vi "PH_Synchrolock_Watch.panel.vi"(0 "object ref":refnum<vi>, 5 "error in (no error)":errorcluster) -> (19 "error out":errorcluster)   [LabVIEW 2014, in "PH_Synchrolock_Watch.lvlib"]
doc: "This a GUI.\n\nLicense Agreement for this software:\n\nCopyright (C)\nGesellschaft für Schwerionenforschung, GSI\nPlanckstr. 1\n64291 Darmstadt\nGermany\n\nContact: D.Beck@gsi.de \n\nThis program is free software; you can redistribute it and/or modify it under the terms of the GNU General Public License as published by the Free Software Foundation; either version 2 of the license, or (at your option) any later version.\n\nThis program is distributed in the hope that it will be useful, but WITHOUT ANYW ARRANTY; without even the implied warranty of MERCHANTABILITY or FITNESS FOR A PARTICULAR PURPOSE. See the GNU General License for more details (http://www.gnu.org).\n\nGesellschaft für Schwerionenforschung, GSI\nPlanckstr. 1, 64291 Darmstadt, Germany\nFor all questions and ideas contact: M.Richter@gsi.de, H.Brand@gsi.de or D.Beck@gsi.de.\nLast update: 18-DEC-2002"
uses:
  PH_Synchrolock_Watch.lvlib
  PH_StatusHandler/PH_StatusHandler.GUI element.ctl
  PH_TKTDS-30xx/PH_TKTDS-30xx.Channel Config.ctl
  PH_TKTDS-30xx/PH_TKTDS-30xx.Acquisition Config.ctl
  PH_TKTDS-30xx/PH_TKTDS-30xx.Trigger Config.ctl
  PH_TKTDS-30xx/PH_TKTDS-30xx.GUI Refs.ctl
  PH_Synchrolock_Watch.Limit to set.ctl
  CSCore/CSObj/CSObj.lvlib
  PH_Common/PH_Common.lvlib
  CSCore/CSSystem/CSSystemLib/CSSystemLib.lvlib
  PH_TKTDS-30xx/PH_TKTDS-30xx.lvlib
  PH_Class/PH_Class.lvlib
  PH_StatusHandler/PH_StatusHandler.lvlib
panel:
  out "VISA Resource":string
  out "Dummy":waveform(dbl)[](graph)
  out "State":u32(colorbox)
  in  "Tab Control":T1(tab)
  in  "Waveform End":i32=10000
  out "MIRA State":u32(colorbox)
  out "Mira scope":cluster{dbl[], dbl[]}[](graph)=[{array[1000 elements], array[1000 elements]}, {array[1000 elements], array[1000 elements]}, {[7.678540433925049e-09, 2.168621418974559e-08, 3.532212428448502e-08, 4.8880103626943005e-08, 6.250409620353807e-08, 7.640981633945535e-08, 9.060849771566783e-08, 1.0463764927718417e-07, 1.1843036179225119e-07, 1.3205722912966255e-07, 1.456689870009999e-07, 1.593456671426305e-07, 1.733563575717145e-07, 1.8748672524777768e-07], [0.1328923695789544, 0.14553699894253908, 0.15804846129472974, 0.158480311601262, 0.15023324530868346, 0.13645178082078474, 0.12443003311658221, 0.1394555004984945, 0.1510217909126647, 0.15823883495688304, 0.1548392047127739, 0.14554396716656443, 0.1297955998863915, 0.1273963557283981]}, {[7.736674157303367e-09, 2.155081885856079e-08, 3.5410718232044194e-08, 4.9320659340659336e-08, 6.315258426966291e-08, 7.696082949308756e-08, 9.076550868486352e-08, 1.045925e-07, 1.1843617486338797e-07, 1.3226125e-07, 1.4617333333333334e-07, 1.6003049180327868e-07, 1.7381259259259259e-07, 1.87644e-07], [0.007461034259448418, 0.0073273846229039786, 0.007350860505608576, 0.006879176956376958, 0.007073457405515834, 0.007321165898617512, 0.0071646017369727056, 0.0071848909090909095, 0.007206295115085282, 0.007172368181818184, 0.007138666666666666, 0.007072396125186293, 0.007497003815937153, 0.007023602424242428]}]
  out "Mean Phase in range?":bool
  out "Mira Amplitude in range?":bool
  out "RF Amplitude above limit?":bool
  in  "Reset Mira warning":bool
  out "Mean Phase Graph":cluster{dbl[], dbl[]}[](graph) caption="Mean Phase"
  out "Mean Phase":dbl=2.090074050465849e-10 caption="Current Value" format="%^#_6e"
  in  "Mean phase upper limit":dbl=0.15 caption="Upper limit" format="%^#_6e"
  in  "Mean phase lower limit":dbl=-0.15 caption="Lower limit" format="%^#_6e"
  out "RF Amplitude Graph":cluster{dbl[], dbl[]}[](graph) caption="RF Amplitude"
  in  "RF Amplitude lower limit":dbl=0.13 caption="Lower limit" format="%^#_6e"
  out "RF Amplitude":dbl=0.14374031818040756 caption="Current Value" format="%^#_6e"
  out "Mira Amplitude Graph":cluster{dbl[], dbl[]}[](graph) caption="Mira Amplitude"
  in  "Mira Amplitude lower limit":dbl=0.0061 caption="Lower limit" format="%^#_6e"
  in  "Mira Amplitude upper limit":dbl=0.0068 caption="Upper limit" format="%^#_6e"
  out "Mira Amplitude":dbl=0.9056406758925662 caption="Current Value" format="%^#_6e"
  in  "Trigger":T2={"Source"="CH1", "Slope"=0, "Level [V]"=0.0} {"Level [V]" format="%#_6p"}
  in  "Acquisition":T3={"Time base"=2e-07, "Record Length"=10000, "Start Time"=0.0, "Type"=0, "Continuous"=FALSE} {"Start Time" format="%#_12p"; "Record Length" items=["500"=500, "10000"=10000]; "Time base" items=["2ns"=2e-09, "4ns"=4e-09, "10ns"=1e-08, "20ns"=2e-08, "40ns"=4e-08, "100ns"=1e-07, "200ns"=2e-07, "400ns"=4e-07, "1µs"=1e-06, "2µs"=2e-06, "4µs"=4e-06, "10µs"=1e-05, "20µs"=2e-05, "40µs"=4e-05, "100µs"=0.0001, "200µs"=0.0002, "400µs"=0.0004, "1ms"=0.001, "2ms"=0.002, "10ms"=0.01, "20ms"=0.02, "40ms"=0.04, "100ms"=0.1, "200ms"=0.2, "400ms"=0.4, "1s"=1.0, "2s"=2.0, "4s"=4.0, "10s"=10.0]}
  in  "Mira Signal":T4={"Channel Name"="CH1", "Input Impedance"="MEG", "Max Input Frequency"="TWENTY", "Vertical Coupling"=1, "Channel Enabled"=TRUE, "Probe Attenuation"=1.0, "Vertical Range"=100.0, "Vertical Offset"=0.0} {"Vertical Offset" format="%#_6p"; "Vertical Range" items=["1mV"=0.001, "2mV"=0.002, "5mV"=0.005, "10mV"=0.01, "20mV"=0.02, "50mV"=0.05, "100mV"=0.1, "200mV"=0.2, "500mV"=0.5, "1V"=1.0]; "Probe Attenuation" format="%#.2f"}
  in  "RF Signal":T4={"Channel Name"="CH1", "Input Impedance"="MEG", "Max Input Frequency"="TWENTY", "Vertical Coupling"=1, "Channel Enabled"=TRUE, "Probe Attenuation"=1.0, "Vertical Range"=100.0, "Vertical Offset"=0.0} {"Vertical Offset" format="%#_6p"; "Vertical Range" items=["1mV"=0.001, "2mV"=0.002, "5mV"=0.005, "10mV"=0.01, "20mV"=0.02, "50mV"=0.05, "100mV"=0.1, "200mV"=0.2, "500mV"=0.5, "1V"=1.0]; "Probe Attenuation" format="%#.2f"}
  in  "Display Intensity":u8=1 min=1 max=100 step=1
  in  "Channel to be positioned":string(combo)="CH1"
  in  "Position":dbl
  out "PSDB Status":u32(colorbox)=6618880 caption="PSDB"
  out "Status":T5 caption="Enabling State"
  in  "Delete":bool
  in  "Exit":bool
  # "PCS"
  # "3.40"
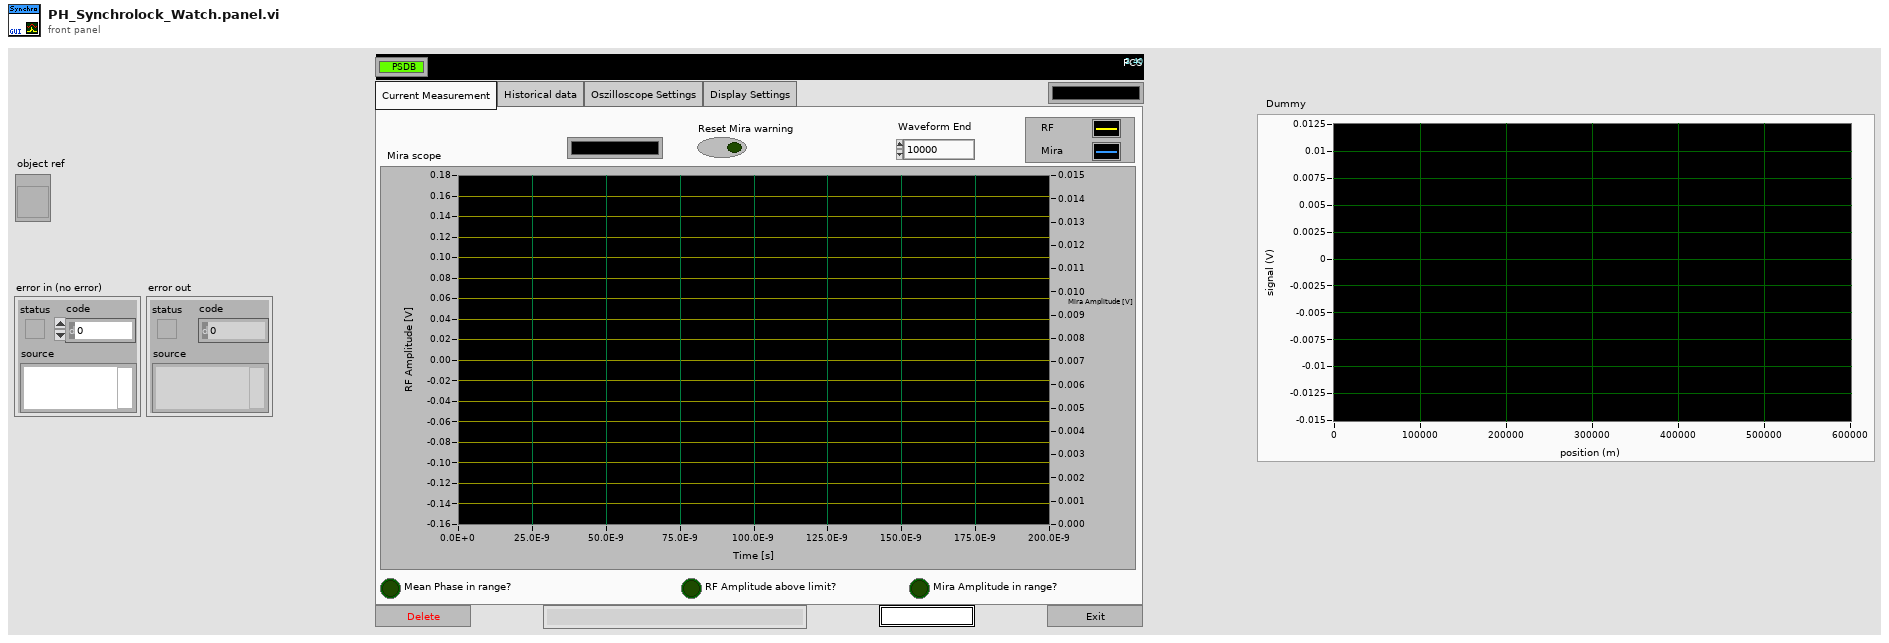
[diagram p1: front panel]
types:
  T1 = enum32{"Current Measurement", "Historical data", "Oszilloscope Settings", "Display Settings"}
  T2 = typedef "PH_TKTDS-30xx.lvlib/PH_TKTDS-30xx.Trigger Config.ctl" = cluster{"Source":string, "Slope":i32, "Level [V]":dbl}
  T3 = typedef "PH_TKTDS-30xx.lvlib/PH_TKTDS-30xx.Acquisition Config.ctl" = cluster{"Time base":dbl, "Record Length":u16, "Start Time":dbl, "Type":i32, "Continuous":bool}
  T4 = typedef "PH_TKTDS-30xx.lvlib/PH_TKTDS-30xx.Channel Config.ctl" = cluster{"Channel Name":string, "Input Impedance":string, "Max Input Frequency":string, "Vertical Coupling":i32, "Channel Enabled":bool, "Probe Attenuation":dbl, "Vertical Range":dbl, "Vertical Offset":dbl}
  T5 = typedef "PH_StatusHandler.lvlib/PH_StatusHandler.GUI element.ctl" = u16
  T6 = typedef "PH_TKTDS-30xx.lvlib/PH_TKTDS-30xx.GUI Refs.ctl" = cluster{"Trigger":refnum<vi>, "Acquisition":refnum<vi>, "Graph":refnum<vi>, "State":refnum<vi>, "Delete":refnum<vi>, "Channel to be positioned":refnum<vi>, "Postion":refnum<vi>, "Display Intensity":refnum<vi>, "VISA Resource":refnum<vi>}
  T7 = cluster{"TEK 30xx GUI Refs":T6, "TEK 30xx Channel Refs":refnum<vi>[], "Ref PSDB Status":refnum<vi>}
  T8 = typedef "PH_Synchrolock_Watch.lvlib/PH_Synchrolock_Watch.Limit to set.ctl" = i16
  T9 = typedef "PH_Synchrolock_Watch.lvlib/PH_Synchrolock_Watch.i attribute.ctl" = cluster{"GUI Refs":cluster{"Mean Phase Graph":refnum<vi>, "RF Amplitude Graph":refnum<vi>, "Mira Amplitude Graph":refnum<vi>, "MIRA State":refnum<vi>, "Mean Phase":refnum<vi>, "RF Amplitude":refnum<vi>, "Mira Amplitude":refnum<vi>, "Mean Phase in range?":refnum<vi>, "RF Amplitude above limit?":refnum<vi>, "Mira Amplitude in range?":refnum<vi>, "Mean phase upper limit":refnum<vi>, "Mean phase lower limit":refnum<vi>, "RF Amplitude lower limit":refnum<vi>, "Mira Amplitude lower limit":refnum<vi>, "Mira Amplitude upper limit":refnum<vi>, "Waveform End":refnum<vi>, "Mira scope":refnum<vi>, "Reset Mira warning":refnum<vi>}, "Status":cluster{"Reset Warning":bool}, "Mean Phase":cluster{"Current Value":dbl, "Upper Limit":dbl, "Lower Limit":dbl, "Data":cluster{dbl[], dbl[]}}, "RF":cluster{"Current Value":dbl, "Lower Limit":dbl, "Data":cluster{dbl[], dbl[]}}, "MIRA":cluster{"Current Value":dbl, "Upper Limit":dbl, "Lower Limit":dbl, "Data":cluster{dbl[], dbl[]}}, "Waveform End":i32}
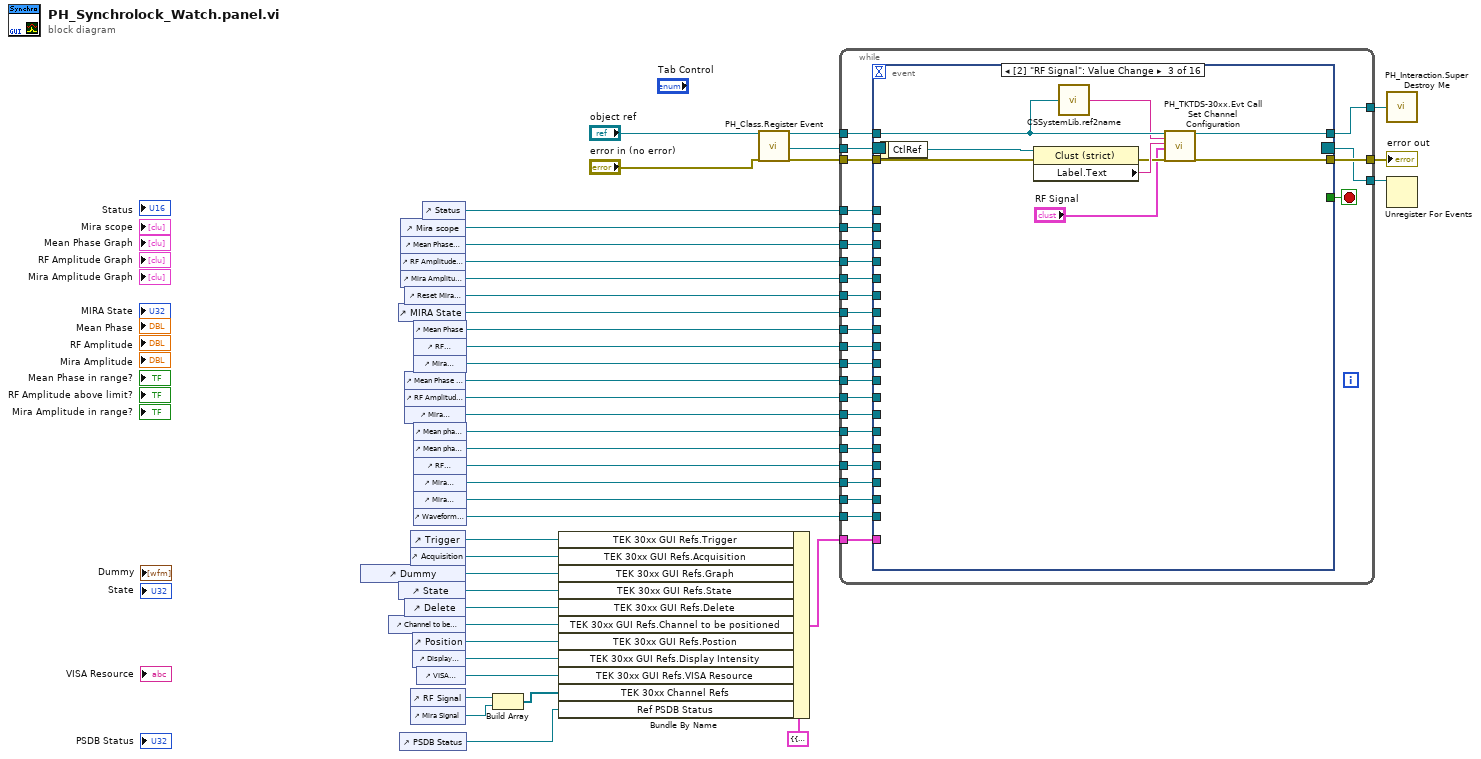
[diagram p0: block diagram]
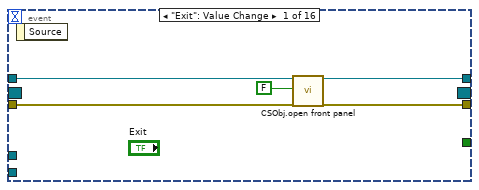
[diagram p2: hidden frame]
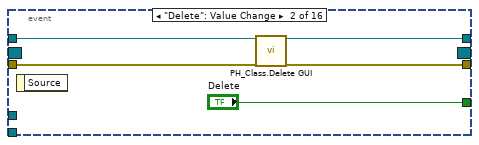
[diagram p3: hidden frame]
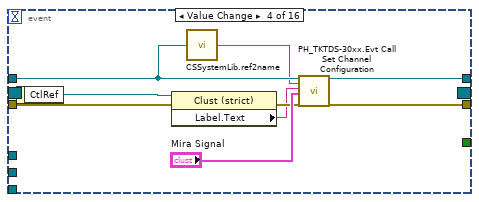
[diagram p4: hidden frame]
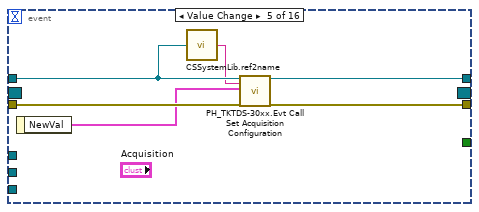
[diagram p5: hidden frame]
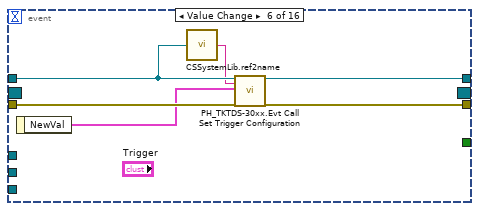
[diagram p6: hidden frame]
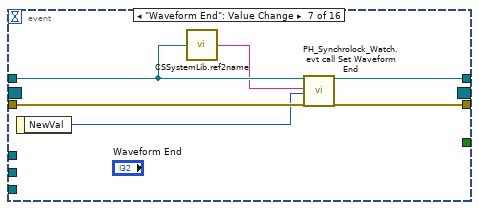
[diagram p7: hidden frame]
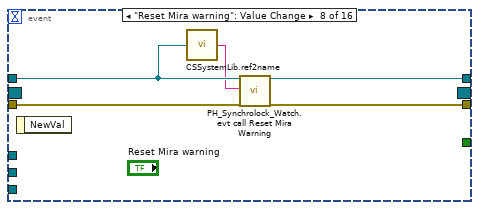
[diagram p8: hidden frame]
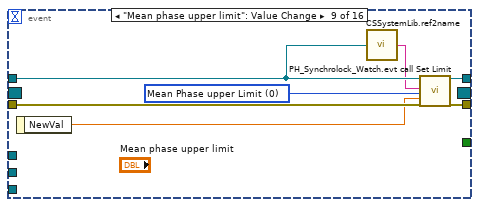
[diagram p9: hidden frame]
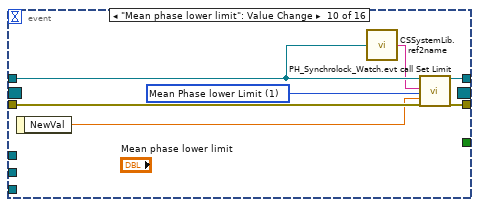
[diagram p10: hidden frame]
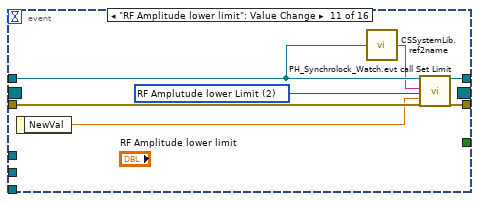
[diagram p11: hidden frame]
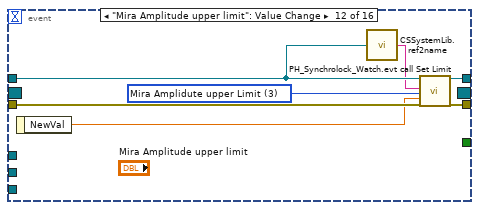
[diagram p12: hidden frame]
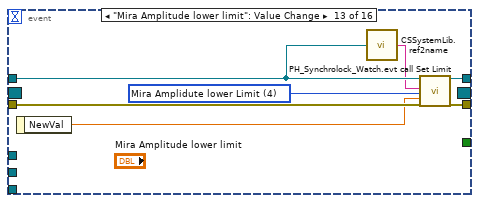
[diagram p13: hidden frame]
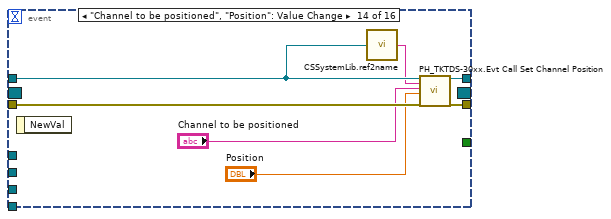
[diagram p14: hidden frame]
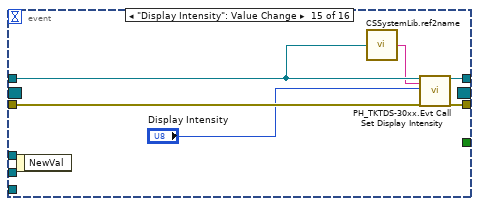
[diagram p15: hidden frame]
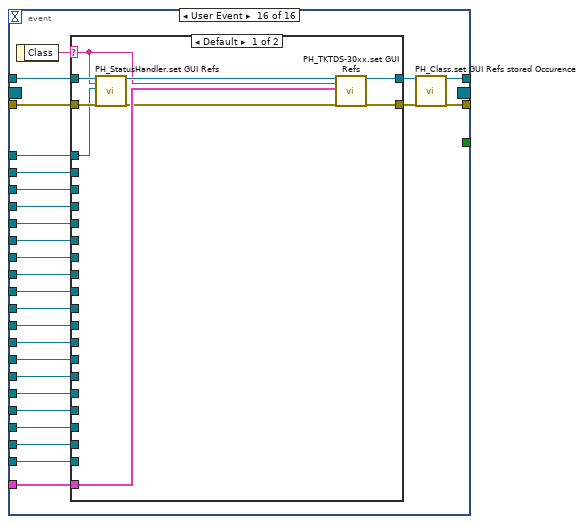
[diagram p16: hidden frame]
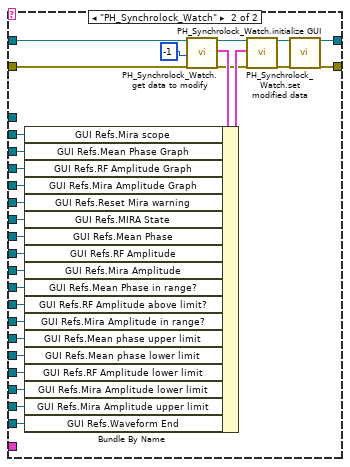
[diagram p17: hidden frame]
diagram:
  n1 = control-ref of="Dummy"() -> (w34:refnum<vi>)
  n2 = control-ref of="Channel to be positioned"() -> (w32:refnum<vi>)
  n3 = control-ref of="MIRA State"() -> (w17:refnum<vi>)
  n4 = control-ref of="State"() -> (w35:refnum<vi>)
  n5 = control-ref of="PSDB Status"() -> (w24:refnum<vi>)
  n6 = control-ref of="Mira scope"() -> (w22:refnum<vi>)
  n7 = control-ref of="Mean Phase Graph"() -> (w21:refnum<vi>)
  n8 = control-ref of="RF Amplitude Graph"() -> (w20:refnum<vi>)
  n9 = control-ref of="Mira Amplitude Graph"() -> (w19:refnum<vi>)
  n10 = control-ref of="Reset Mira warning"() -> (w18:refnum<vi>)
  n11 = control-ref of="Mean Phase in range?"() -> (w13:refnum<vi>)
  n12 = control-ref of="RF Amplitude above limit?"() -> (w12:refnum<vi>)
  n13 = control-ref of="Mira Amplitude in range?"() -> (w11:refnum<vi>)
  n14 = control-ref of="Delete"() -> (w38:refnum<vi>)
  n15 = control-ref of="Trigger"() -> (w37:refnum<vi>)
  n16 = control-ref of="Acquisition"() -> (w36:refnum<vi>)
  n17 = control-ref of="RF Signal"() -> (w40:refnum<vi>)
  n18 = control-ref of="Mira Signal"() -> (w39:refnum<vi>)
  n19 = control-ref of="Position"() -> (w31:refnum<vi>)
  n20 = control-ref of="Display Intensity"() -> (w33:refnum<vi>)
  n21 = control-ref of="Mean Phase"() -> (w16:refnum<vi>)
  n22 = control-ref of="RF Amplitude"() -> (w15:refnum<vi>)
  n23 = control-ref of="Mira Amplitude"() -> (w14:refnum<vi>)
  n24 = control-ref of="Mean phase upper limit"() -> (w10:refnum<vi>)
  n25 = control-ref of="Mean phase lower limit"() -> (w9:refnum<vi>)
  n26 = control-ref of="RF Amplitude lower limit"() -> (w8:refnum<vi>)
  n27 = control-ref of="Mira Amplitude lower limit"() -> (w7:refnum<vi>)
  n28 = control-ref of="Mira Amplitude upper limit"() -> (w6:refnum<vi>)
  n29 = control-ref of="Waveform End"() -> (w5:refnum<vi>)
  n30 = control-ref of="VISA Resource"() -> (w30:refnum<vi>)
  n31 = control-ref of="Status"() -> (w1:refnum<vi>)
  n32 = Build Array(w40, w39) -> (w23:refnum<vi>[])
  n33 = Bundle By Name(cluster=T7 {"TEK 30xx GUI Refs"={"Trigger"=refnum, "Acquisition"=refnum, "Graph"=refnum, "State"=refnum, "Delete"=refnum, "Channel to be positioned"=refnum, "Postion"=refnum, "Display Intensity"=refnum, "VISA Resource"=refnum}, "TEK 30xx Channel Refs"=[], "Ref PSDB Status"=refnum} ("GUI Refs"), "TEK 30xx GUI Refs.Trigger"=w37, "TEK 30xx GUI Refs.Acquisition"=w36, "TEK 30xx GUI Refs.Graph"=w34, "TEK 30xx GUI Refs.State"=w35, "TEK 30xx GUI Refs.Delete"=w38, "TEK 30xx GUI Refs.Channel to be positioned"=w32, "TEK 30xx GUI Refs.Postion"=w31, "TEK 30xx GUI Refs.Display Intensity"=w33, "TEK 30xx GUI Refs.VISA Resource"=w30, "TEK 30xx Channel Refs"=w23, "Ref PSDB Status"=w24) -> (w4:T7)
  n34 = call "PH_Class.Register Event.vi"("i ref in"="object ref", "error in (no error)"="error in (no error)") -> ("i ref out"=w29:refnum<vi>, "Event Registration Refnum"=w27:refnum<event-registration>, "error out"=w28:errorcluster)  [unwired: 15 in]
  n35 = while {
    tunnel: w29 -> [w66]
    tunnel: [w65] -> w42
    tunnel: w28 -> [w68]
    tunnel: [w67] -> w41
    tunnel: w27 -> [w64]
    tunnel: [w63] -> w26
    tunnel: w1 -> [w62]
    tunnel: w22 -> [w61]
    tunnel: w21 -> [w60]
    tunnel: w20 -> [w59]
    tunnel: w19 -> [w58]
    tunnel: w18 -> [w57]
    tunnel: w17 -> [w56]
    tunnel: w16 -> [w55]
    tunnel: w15 -> [w54]
    tunnel: w14 -> [w53]
    tunnel: w13 -> [w52]
    tunnel: w12 -> [w51]
    tunnel: w11 -> [w50]
    tunnel: w10 -> [w49]
    tunnel: w9 -> [w48]
    tunnel: w8 -> [w47]
    tunnel: w7 -> [w46]
    tunnel: w6 -> [w45]
    tunnel: w5 -> [w44]
    tunnel: w4 -> [w43]
    stop <- w69 stop-if-true
    n36 = event shown="[2] \"RF Signal\": Value Change" {
      selector: w64 -> [_ _ _ _ _ _ _ _ _ _ _ _ _ _ _ _]
      dyn-events: [_ _ _ _ _ _ _ _ _ _ _ _ _ _ _ _] -> w63
      timeout: _ -> [_ _ _ _ _ _ _ _ _ _ _ _ _ _ _ _]
      tunnel: [_ "Delete" _ _ _ _ _ _ _ _ _ _ _ _ _ _] -> w69
      tunnel: w66 -> [w71 w76 w86 w95 w100 w106 w112 w117 w124 w131 w138 w145 w152 w159 w165 w193]
      tunnel: w68 -> [w74 w78 w82 w90 w103 w109 w115 w120 w127 w134 w141 w148 w155 w162 w168 w192]
      tunnel: [w73 w77 w88 w97 w102 w108 w114 w119 w126 w133 w140 w147 w154 w161 w167 w194] -> w67
      tunnel: [w70 w75 w87 w96 w101 w107 w113 w118 w125 w132 w139 w146 w153 w160 w166 w195] -> w65
      tunnel: w62 -> [_ _ _ _ _ _ _ _ _ _ _ _ _ _ _ w189]
      tunnel: w61 -> [_ _ _ _ _ _ _ _ _ _ _ _ _ _ _ w188]
      tunnel: w60 -> [_ _ _ _ _ _ _ _ _ _ _ _ _ _ _ w187]
      tunnel: w59 -> [_ _ _ _ _ _ _ _ _ _ _ _ _ _ _ w186]
      tunnel: w58 -> [_ _ _ _ _ _ _ _ _ _ _ _ _ _ _ w185]
      tunnel: w57 -> [_ _ _ _ _ _ _ _ _ _ _ _ _ _ _ w184]
      tunnel: w56 -> [_ _ _ _ _ _ _ _ _ _ _ _ _ _ _ w183]
      tunnel: w55 -> [_ _ _ _ _ _ _ _ _ _ _ _ _ _ _ w182]
      tunnel: w54 -> [_ _ _ _ _ _ _ _ _ _ _ _ _ _ _ w181]
      tunnel: w53 -> [_ _ _ _ _ _ _ _ _ _ _ _ _ _ _ w180]
      tunnel: w52 -> [_ _ _ _ _ _ _ _ _ _ _ _ _ _ _ w179]
      tunnel: w51 -> [_ _ _ _ _ _ _ _ _ _ _ _ _ _ _ w178]
      tunnel: w50 -> [_ _ _ _ _ _ _ _ _ _ _ _ _ _ _ w177]
      tunnel: w49 -> [_ _ _ _ _ _ _ _ _ _ _ _ _ _ _ w176]
      tunnel: w48 -> [_ _ _ _ _ _ _ _ _ _ _ _ _ _ _ w175]
      tunnel: w47 -> [_ _ _ _ _ _ _ _ _ _ _ _ _ _ _ w174]
      tunnel: w46 -> [_ _ _ _ _ _ _ _ _ _ _ _ _ _ _ w173]
      tunnel: w45 -> [_ _ _ _ _ _ _ _ _ _ _ _ _ _ _ w172]
      tunnel: w44 -> [_ _ _ _ _ _ _ _ _ _ _ _ _ _ _ w171]
      tunnel: w43 -> [_ _ _ _ _ _ _ _ _ _ _ _ _ _ _ w169]
      event "Exit": Value Change {
        n37 = event-data() -> ()  [unwired: 1 in, 1 out]
        n38 = call "CSObj.open front panel.vi"("i ref in"=w71, "frontPanelOpen"=FALSE ("front panel open"), "error in (no error)"=w74) -> ("i ref out"=w70:refnum<vi>, "error out"=w73:errorcluster)  [unwired: 15 in]
      }
      event "Delete": Value Change {
        n39 = event-data() -> ()  [unwired: 1 in, 1 out]
        n40 = call "PH_Class.Delete GUI.vi"("VI in"=w76, "error in (no error)"=w78) -> ("VI out"=w75:refnum<vi>, "error out"=w77:errorcluster)  [unwired: 16 in]
      }
      event Value Change {
        n41 = event-data() -> ("CtlRef"=w85:refnum<vi>)  [unwired: 1 in]
        n42 = property class="Clust (strict)"(reference=w85, error in=w82) -> (error out=w81:errorcluster, "Label.Text"=w83:string)  [unwired: 1 out]
        n43 = call "CSSystemLib.ref2name.vi"("obj refnum"=w86) -> ("name"=w84:string)
        n44 = call "PH_TKTDS-30xx.Evt Call Set Channel Configuration.vi"("i ref in"=w86, "Instance"=w84, "GUI Element Name"=w83, "Channel Configuration"="RF Signal", "error in (no error)"=w81) -> ("i ref out"=w87:refnum<vi>, "error out"=w88:errorcluster)  [unwired: 13 in]
      }
      event Value Change {
        n45 = event-data() -> ("CtlRef"=w92:refnum<vi>)  [unwired: 1 in]
        n46 = property class="Clust (strict)"(reference=w92, error in=w90) -> (error out=w91:errorcluster, "Label.Text"=w89:string)  [unwired: 1 out]
        n47 = call "CSSystemLib.ref2name.vi"("obj refnum"=w95) -> ("name"=w94:string)
        n48 = call "PH_TKTDS-30xx.Evt Call Set Channel Configuration.vi"("i ref in"=w95, "Instance"=w94, "GUI Element Name"=w89, "Channel Configuration"="Mira Signal", "error in (no error)"=w91) -> ("i ref out"=w96:refnum<vi>, "error out"=w97:errorcluster)  [unwired: 13 in]
      }
      event Value Change {
        n49 = event-data() -> ("NewVal"=w98:T3)  [unwired: 1 in]
        n50 = call "CSSystemLib.ref2name.vi"("obj refnum"=w100) -> ("name"=w99:string)
        n51 = call "PH_TKTDS-30xx.Evt Call Set Acquisition Configuration.vi"("i ref in"=w100, "Instance"=w99, "Acquisition Configuration"=w98, "error in (no error)"=w103) -> ("i ref out"=w101:refnum<vi>, "error out"=w102:errorcluster)  [unwired: 14 in]
      }
      event Value Change {
        n52 = event-data() -> ("NewVal"=w104:T2)  [unwired: 1 in]
        n53 = call "CSSystemLib.ref2name.vi"("obj refnum"=w106) -> ("name"=w105:string)
        n54 = call "PH_TKTDS-30xx.Evt Call Set Trigger Configuration.vi"("i ref in"=w106, "Instance"=w105, "Trigger Configuration"=w104, "error in (no error)"=w109) -> ("i ref out"=w107:refnum<vi>, "error out"=w108:errorcluster)  [unwired: 14 in]
      }
      event "Waveform End": Value Change {
        n55 = event-data() -> ("NewVal"=w110:i32)  [unwired: 1 in]
        n56 = call "CSSystemLib.ref2name.vi"("obj refnum"=w112) -> ("name"=w111:string)
        n57 = call "PH_Synchrolock_Watch.evt call Set Waveform End.vi"("i ref in"=w112, "Instance"=w111, "Waveform End"=w110, "error in (no error)"=w115) -> ("i ref out"=w113:refnum<vi>, "error out"=w114:errorcluster)  [unwired: 14 in]
      }
      event "Reset Mira warning": Value Change {
        n58 = event-data() -> ()  [unwired: 1 in, 1 out]
        n59 = call "CSSystemLib.ref2name.vi"("obj refnum"=w117) -> ("name"=w116:string)
        n60 = call "PH_Synchrolock_Watch.evt call Reset Mira Warning.vi"("i ref in"=w117, "Instance"=w116, "error in (no error)"=w120) -> ("i ref out"=w118:refnum<vi>, "error out"=w119:errorcluster)  [unwired: 15 in]
      }
      event "Mean phase upper limit": Value Change {
        w121 = T8 0 items=["Mean Phase upper Limit", "Mean Phase lower Limit", "RF Amplutude lower Limit", "Mira Amplidute upper Limit", "Mira Amplidute lower Limit"] ("Limit to set")
        n61 = event-data() -> ("NewVal"=w122:dbl)  [unwired: 1 in]
        n62 = call "CSSystemLib.ref2name.vi"("obj refnum"=w124) -> ("name"=w123:string)
        n63 = call "PH_Synchrolock_Watch.evt call Set Limit.vi"("i ref in"=w124, "Instance"=w123, "Limit to set"=w121, "Limit"=w122, "error in (no error)"=w127) -> ("i ref out"=w125:refnum<vi>, "error out"=w126:errorcluster)  [unwired: 13 in]
      }
      event "Mean phase lower limit": Value Change {
        w128 = T8 1 items=["Mean Phase upper Limit", "Mean Phase lower Limit", "RF Amplutude lower Limit", "Mira Amplidute upper Limit", "Mira Amplidute lower Limit"] ("Limit to set")
        n64 = event-data() -> ("NewVal"=w129:dbl)  [unwired: 1 in]
        n65 = call "CSSystemLib.ref2name.vi"("obj refnum"=w131) -> ("name"=w130:string)
        n66 = call "PH_Synchrolock_Watch.evt call Set Limit.vi"("i ref in"=w131, "Instance"=w130, "Limit to set"=w128, "Limit"=w129, "error in (no error)"=w134) -> ("i ref out"=w132:refnum<vi>, "error out"=w133:errorcluster)  [unwired: 13 in]
      }
      event "RF Amplitude lower limit": Value Change {
        w135 = T8 2 items=["Mean Phase upper Limit", "Mean Phase lower Limit", "RF Amplutude lower Limit", "Mira Amplidute upper Limit", "Mira Amplidute lower Limit"] ("Limit to set")
        n67 = event-data() -> ("NewVal"=w136:dbl)  [unwired: 1 in]
        n68 = call "CSSystemLib.ref2name.vi"("obj refnum"=w138) -> ("name"=w137:string)
        n69 = call "PH_Synchrolock_Watch.evt call Set Limit.vi"("i ref in"=w138, "Instance"=w137, "Limit to set"=w135, "Limit"=w136, "error in (no error)"=w141) -> ("i ref out"=w139:refnum<vi>, "error out"=w140:errorcluster)  [unwired: 13 in]
      }
      event "Mira Amplitude upper limit": Value Change {
        w142 = T8 3 items=["Mean Phase upper Limit", "Mean Phase lower Limit", "RF Amplutude lower Limit", "Mira Amplidute upper Limit", "Mira Amplidute lower Limit"] ("Limit to set")
        n70 = event-data() -> ("NewVal"=w143:dbl)  [unwired: 1 in]
        n71 = call "CSSystemLib.ref2name.vi"("obj refnum"=w145) -> ("name"=w144:string)
        n72 = call "PH_Synchrolock_Watch.evt call Set Limit.vi"("i ref in"=w145, "Instance"=w144, "Limit to set"=w142, "Limit"=w143, "error in (no error)"=w148) -> ("i ref out"=w146:refnum<vi>, "error out"=w147:errorcluster)  [unwired: 13 in]
      }
      event "Mira Amplitude lower limit": Value Change {
        w149 = T8 4 items=["Mean Phase upper Limit", "Mean Phase lower Limit", "RF Amplutude lower Limit", "Mira Amplidute upper Limit", "Mira Amplidute lower Limit"] ("Limit to set")
        n73 = event-data() -> ("NewVal"=w150:dbl)  [unwired: 1 in]
        n74 = call "CSSystemLib.ref2name.vi"("obj refnum"=w152) -> ("name"=w151:string)
        n75 = call "PH_Synchrolock_Watch.evt call Set Limit.vi"("i ref in"=w152, "Instance"=w151, "Limit to set"=w149, "Limit"=w150, "error in (no error)"=w155) -> ("i ref out"=w153:refnum<vi>, "error out"=w154:errorcluster)  [unwired: 13 in]
      }
      event "Channel to be positioned", "Position": Value Change {
        n76 = event-data() -> ()  [unwired: 1 in, 1 out]
        n77 = call "CSSystemLib.ref2name.vi"("obj refnum"=w159) -> ("name"=w158:string)
        n78 = call "PH_TKTDS-30xx.Evt Call Set Channel Position.vi"("i ref in"=w159, "Instance"=w158, "Channel to be positioned"="Channel to be positioned", "Position"="Position", "error in (no error)"=w162) -> ("i ref out"=w160:refnum<vi>, "error out"=w161:errorcluster)  [unwired: 13 in]
      }
      event "Display Intensity": Value Change {
        n79 = event-data() -> ()  [unwired: 1 in, 1 out]
        n80 = call "CSSystemLib.ref2name.vi"("obj refnum"=w165) -> ("name"=w164:string)
        n81 = call "PH_TKTDS-30xx.Evt Call Set Display Intensity.vi"("i ref in"=w165, "Instance"=w164, "Display Intensity"="Display Intensity", "error in (no error)"=w168) -> ("i ref out"=w166:refnum<vi>, "error out"=w167:errorcluster)  [unwired: 14 in]
      }
      event User Event {
        n82 = event-data() -> ("Class"=w170:string)  [unwired: 1 in]
        n83 = case shown="Default" w170 {
          selector: w170 -> [w197 _]
          tunnel: w193 -> [w199 w228]
          tunnel: w192 -> [w204 w227]
          tunnel: [w203 w206] -> w191
          tunnel: [w202 w205] -> w190
          tunnel: w189 -> [w196 _]
          tunnel: w188 -> [_ w226]
          tunnel: w187 -> [_ w225]
          tunnel: w186 -> [_ w224]
          tunnel: w185 -> [_ w223]
          tunnel: w184 -> [_ w222]
          tunnel: w183 -> [_ w221]
          tunnel: w182 -> [_ w220]
          tunnel: w181 -> [_ w219]
          tunnel: w180 -> [_ w218]
          tunnel: w179 -> [_ w217]
          tunnel: w178 -> [_ w216]
          tunnel: w177 -> [_ w215]
          tunnel: w176 -> [_ w214]
          tunnel: w175 -> [_ w213]
          tunnel: w174 -> [_ w212]
          tunnel: w173 -> [_ w211]
          tunnel: w172 -> [_ w210]
          tunnel: w171 -> [_ w209]
          tunnel: w169 -> [w201 _]
          frame Default {
            n84 = call "PH_StatusHandler.set GUI Refs.vi"("i ref in"=w199, "Class"=w197, "GUI Ref"=w196, "error in (no error)"=w204) -> ("i ref out"=w198:refnum<vi>, "error out"=w200:errorcluster)  [unwired: 14 in]
            n85 = call "PH_TKTDS-30xx.set GUI Refs.vi"("i ref in"=w198, "Class"=w197, "GUI Refs"=w201, "error in (no error)"=w200) -> ("i ref out"=w203:refnum<vi>, "error out"=w202:errorcluster)  [unwired: 14 in]
          }
          frame "PH_Synchrolock_Watch" {
            n86 = call "PH_Synchrolock_Watch.get data to modify.vi"("i ref in"=w228, "ms timeout (10000)"=-1, "error in (no error)"=w227) -> ("i ref out"=w229:refnum<vi>, "i attribute"=w231:T9, "error out"=w230:errorcluster)  [unwired: 13 in, 1 out]
            n87 = Bundle By Name(cluster=w231, "GUI Refs.Mira scope"=w226, "GUI Refs.Mean Phase Graph"=w225, "GUI Refs.RF Amplitude Graph"=w224, "GUI Refs.Mira Amplitude Graph"=w223, "GUI Refs.Reset Mira warning"=w222, "GUI Refs.MIRA State"=w221, "GUI Refs.Mean Phase"=w220, "GUI Refs.RF Amplitude"=w219, "GUI Refs.Mira Amplitude"=w218, "GUI Refs.Mean Phase in range?"=w217, "GUI Refs.RF Amplitude above limit?"=w216, "GUI Refs.Mira Amplitude in range?"=w215, "GUI Refs.Mean phase upper limit"=w214, "GUI Refs.Mean phase lower limit"=w213, "GUI Refs.RF Amplitude lower limit"=w212, "GUI Refs.Mira Amplitude lower limit"=w211, "GUI Refs.Mira Amplitude upper limit"=w210, "GUI Refs.Waveform End"=w209) -> (w232:T9)
            n88 = call "PH_Synchrolock_Watch.set modified data.vi"("i ref in"=w229, "i attribute"=w232, "error in (no error)"=w230) -> ("i ref out"=w207:refnum<vi>, "error out"=w208:errorcluster)  [unwired: 15 in]
            n89 = call "PH_Synchrolock_Watch.initialize GUI.vi"("i ref in"=w207, "error in (no error)"=w208) -> ("i ref out"=w206:refnum<vi>, "error out"=w205:errorcluster)  [unwired: 16 in]
          }
        }
        n90 = call "PH_Class.set GUI Refs stored Occurence.vi"("i ref in"=w191, "error in (no error)"=w190) -> ("i ref out"=w195:refnum<vi>, "error out"=w194:errorcluster)  [unwired: 16 in]
      }
    }
  }
  "error out" <- w41
  n91 = call "PH_Interaction.Super Destroy Me.vi"("i ref out"=w42) -> ()
  n92 = Unregister For Events(event registration refnum=w26) -> ()  [unwired: 1 in, 1 out]
